vi "clip_number.vi"(9 "x":dbl(slide) min=-1000.0 max=1000.0 scale=-1000.0..1000.0, 10 "lower limit":dbl, 11 "upper limit":dbl) -> (2 "x-y":dbl)   [LabVIEW 2019]
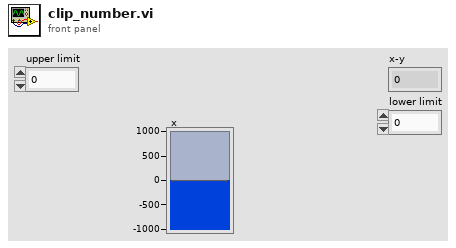
[diagram p1: front panel]
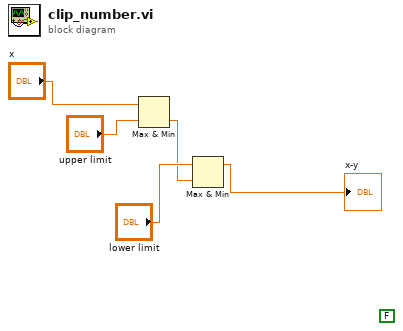
[diagram p0: block diagram]
diagram:
  (unwired) FALSE
  n1 = Max & Min(x="x", y="upper limit") -> (min(x,y)=w3:dbl)  [unwired: 1 out]
  n2 = Max & Min(x="lower limit", y=w3) -> (max(x,y)=→"x-y":dbl)  [unwired: 1 out]
